vi "Division2.vi"(7 "Scale_select":u32=1, 8 "error in (no error)":errorcluster, 9 "V/div":dbl, 10 "s/div":dbl, 11 "WaveformGraph in":refnum<vi>) -> (0 "error out":errorcluster, 2 "V/DIV":string, 3 "S/DIV":string)   [LabVIEW 2019]
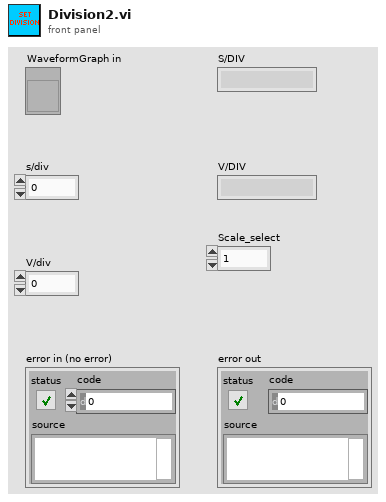
[diagram p1: front panel]
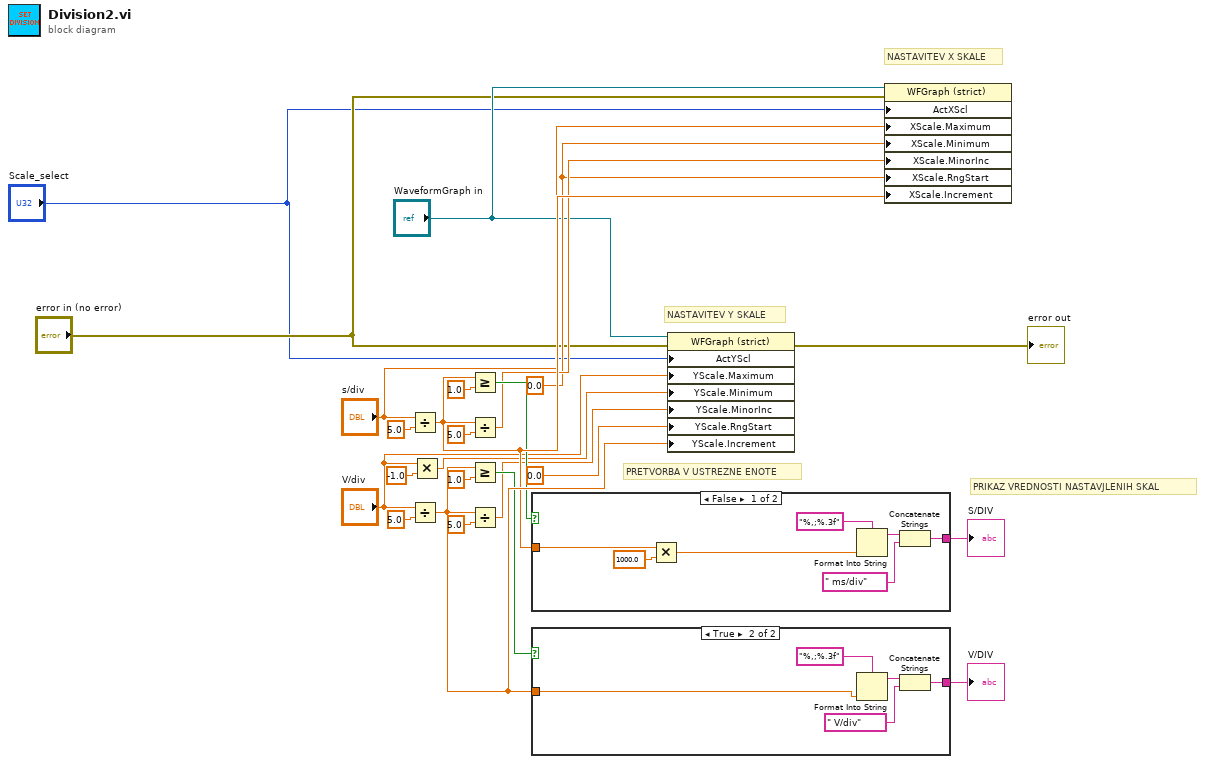
[diagram p0: block diagram]
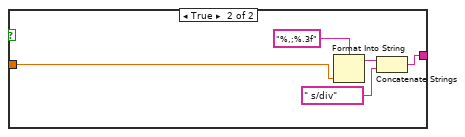
[diagram p2: hidden frame]
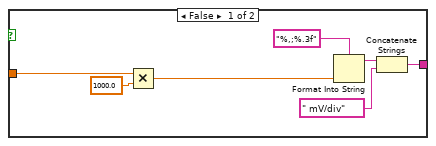
[diagram p3: hidden frame]
diagram:
  w14 = 0.0 ("X Scale.Range:Minimum")
  # "PRETVORBA V USTREZNE ENOTE"
  # "PRIKAZ VREDNOSTI NASTAVJLENIH SKAL"
  # "NASTAVITEV Y SKALE"
  # "NASTAVITEV X SKALE"
  n1 = Divide(x="s/div", y=5.0) -> (x/y=w21:dbl)
  n2 = Divide(x="V/div", y=5.0) -> (x/y=w22:dbl)
  n3 = Multiply(x="V/div", y=-1.0 ("X Scale.Range:Minimum")) -> (x*y=w9:dbl)
  n4 = Greater Or Equal?(x=w21, y=1.0) -> (x >= y?=w19:bool)
  n5 = Divide(x=w21, y=5.0 ("X Scale.Range:Minimum")) -> (x/y=w15:dbl)
  n6 = Greater Or Equal?(x=w22, y=1.0) -> (x >= y?=w18:bool)
  n7 = Divide(x=w22, y=5.0 ("X Scale.Range:Minimum")) -> (x/y=w11:dbl)
  n8 = case shown="False" w19 {
    tunnel: [w26 w34] -> w23
    tunnel: w21 -> [w25 w32]
    frame False {
      n9 = Multiply(x=w25, y=1000.0) -> (x*y=w27:dbl)
      n10 = Format Into String(format string="%,;%.3f", w27) -> (resulting string=w30:string)  [unwired: 2 in, 1 out]
      n11 = Concatenate Strings(w30, " ms/div") -> (w26:string)
    }
    frame True {
      n12 = Format Into String(format string="%,;%.3f", w32) -> (resulting string=w33:string)  [unwired: 2 in, 1 out]
      n13 = Concatenate Strings(w33, " s/div") -> (w34:string)
    }
  }
  "S/DIV" <- w23
  n14 = case shown="True" w18 {
    tunnel: [w38 w46] -> w24
    tunnel: w22 -> [w37 w44]
    frame False {
      n15 = Multiply(x=w37, y=1000.0) -> (x*y=w39:dbl)
      n16 = Format Into String(format string="%,;%.3f", w39) -> (resulting string=w42:string)  [unwired: 2 in, 1 out]
      n17 = Concatenate Strings(w42, " mV/div") -> (w38:string)
    }
    frame True {
      n18 = Format Into String(format string="%,;%.3f", w44) -> (resulting string=w45:string)  [unwired: 2 in, 1 out]
      n19 = Concatenate Strings(w45, " V/div") -> (w46:string)
    }
  }
  "V/DIV" <- w24
  n20 = property on="Property Node" class="WFGraph (strict)"(reference="WaveformGraph in", error in="error in (no error)", "ActYScl"="Scale_select", "YScale.Maximum"="V/div", "YScale.Minimum"=w9, "YScale.MinorInc"=w11, "YScale.RngStart"=0.0 ("X Scale.Range:Minimum"), "YScale.Increment"=w22) -> (error out=→"error out":errorcluster)  [unwired: 1 out]
  n21 = property on="Property Node" class="WFGraph (strict)"(reference="WaveformGraph in", error in="error in (no error)", "ActXScl"="Scale_select", "XScale.Maximum"="s/div", "XScale.Minimum"=w14, "XScale.MinorInc"=w15, "XScale.RngStart"=w14, "XScale.Increment"=w21) -> ()  [unwired: 2 out]
